vi "Sequence MAXMINvalue set.vi"(7 "Channel  (1: CH1)":u16(ring)=1 items=["CH1"=1, "CH2"=2, "CH3"=3, "CH4"=4], 8 "error in (no error)":errorcluster, 9 "MIN":dbl, 10 "MAX":dbl, 11 "VISA resource name":refnum<visa-resource-name>) -> (0 "error out":errorcluster, 3 "VISA resource name out":refnum<visa-resource-name>)   [LabVIEW 2020, in "GPP.lvlib"]
uses:
  GPP.lvlib
  Function/VISA_COMMON.ctl
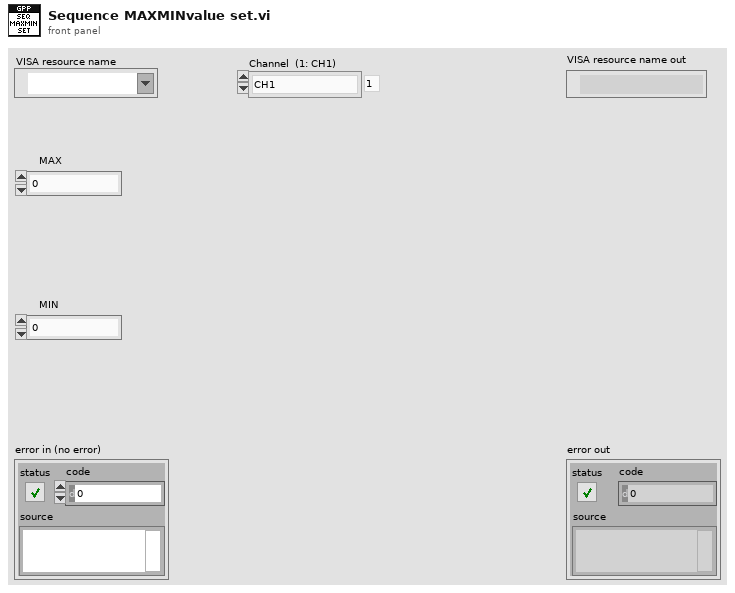
[diagram p1: front panel]
types:
  T1 = typedef "GPP.lvlib/VISA_COMMON.ctl" = enum16{"Initial", "Write CMD", "Read Result", "Read History", "Close"}
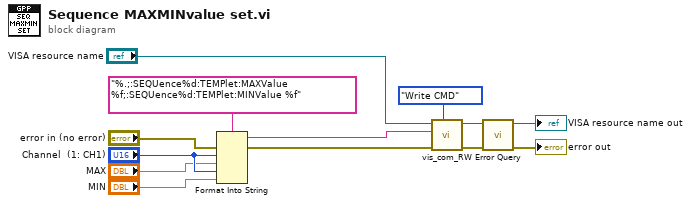
[diagram p0: block diagram]
diagram:
  n1 = Format Into String(format string="%.;:SEQUence%d:TEMPlet:MAXValue %f;:SEQUence%d:TEMPlet:MINValue %f", error in="error in (no error)", "Channel  (1: CH1)", "MAX", "Channel  (1: CH1)", "MIN") -> (resulting string=w1:string, error out=w7:errorcluster)  [unwired: 1 in]
  n2 = call "vis_com_RW.vi"("Funciton"=VISA_COMMON."Write CMD", "error in (no error)"=w7, "CMD String"=w1, "VISA resource in"="VISA resource name") -> ("error out"=w9:errorcluster, "VISA resource out"=w8:refnum<visa-resource-name>)  [unwired: 5 in, 1 out]
  n3 = call "Error Query.vi"("error in (no error)"=w9, "VISA resource name"=w8) -> ("error out"=→"error out":errorcluster, "VISA resource name out"=→"VISA resource name out":refnum<visa-resource-name>)  [unwired: 6 in, 2 out]
